vi "Barcode Printer Port.vi"(10 "string to write":string="I8,A\nq544\nS2\nO\nJF\nWN\nZT\nQ160,25\nN\nb22,31,D,c22,r22,h5,\"0607AA0461NTDB050CT120506TIT00000001\"\nA517,142,2,4,1,1,N,\"M&M:0607AP0461N\"\nA518,117,2,4,1,1,N,\"00000601\"\nA518,92,2,4,1,1,N,\"DA050C\"\nA378,117,2,4,1,1,N,\"120501 I\"\nA518,66,2,4,1,1,N,\"MI:BD07 29049259 BR9.5\"\nP1\n") -> (1 "error out":errorcluster)   [LabVIEW 2020]
uses:
  MS SQL/MS_Global.vi
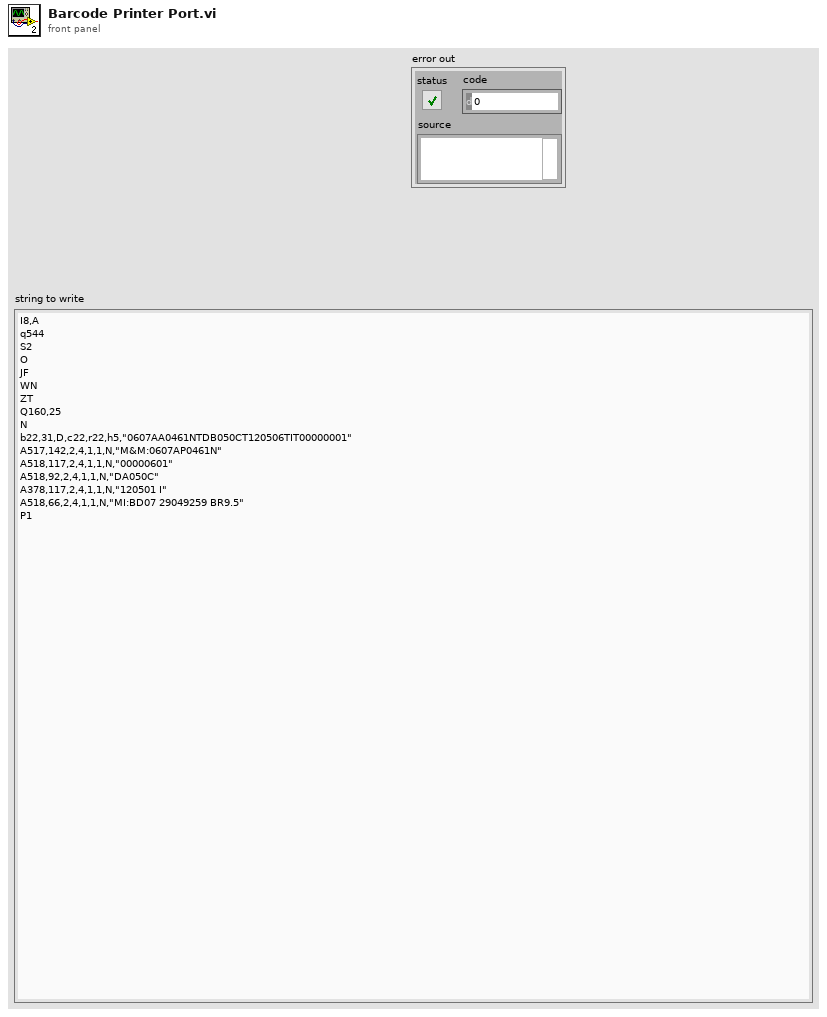
[diagram p1: front panel]
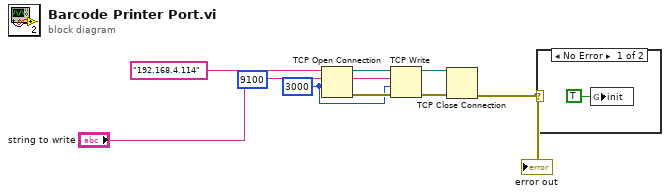
[diagram p0: block diagram]
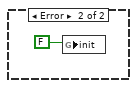
[diagram p2: hidden frame]
diagram:
  w4 = 3000 ("timeout ms (60000)")
  n1 = TCP Open Connection(address="192.168.4.114", remote port or service name=u16 9100, timeout ms (60000)=w4) -> (connection ID=w6:refnum<k5>, error out=w5:errorcluster)  [unwired: 2 in]
  n2 = TCP Write(connection ID=w6, data in="string to write", error in (no error)=w5, 9:w4) -> (connection ID out=w2:refnum<k5>, error out=w3:errorcluster)  [unwired: 1 out]
  n3 = TCP Close Connection(connection ID=w2, error in (no error)=w3) -> (error out=w1:errorcluster)  [unwired: 1 in, 1 out]
  "error out" <- w1
  n4 = case shown="No Error" w1 {
    frame No Error {
      n5 = global write "MS_Global.vi" "init"(TRUE ("init")) -> ()
    }
    frame Error {
      n6 = global write "MS_Global.vi" "init"(FALSE ("init")) -> ()
    }
  }
